vi "Write Max Redirects.vi"(8 "error in (no error)":errorcluster, 10 "max redirects (-1 = no limit)":i32=-1, 11 "REST Client in":refnum<class "REST Client.lvclass">) -> (0 "error out":errorcluster, 3 "REST Client out":refnum<class "REST Client.lvclass">)   [LabVIEW 2020, in "REST Client.lvlib" / "REST Client.lvclass"]
uses:
  REST Client.lvclass
  REST Client.lvclass/REST Client.ctl
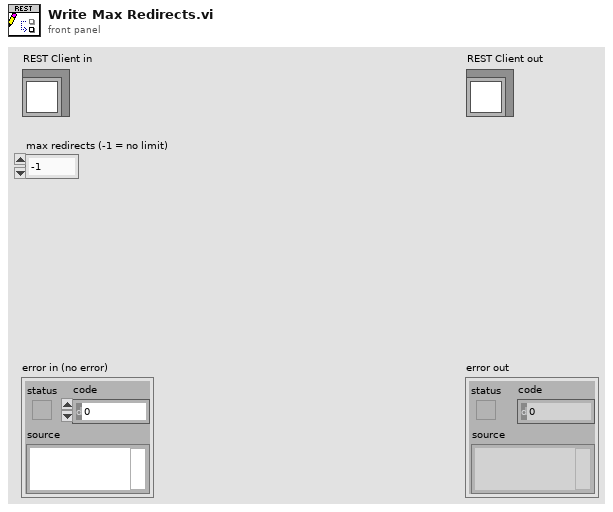
[diagram p1: front panel]
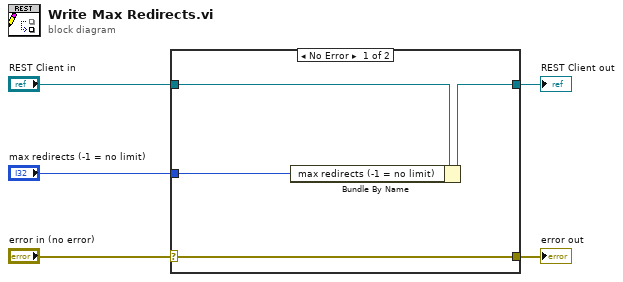
[diagram p0: block diagram]
diagram:
  n1 = case shown="No Error" "error in (no error)" {
    selector: "error in (no error)" -> [w9 w10]
    tunnel: [w9 w10] -> w4
    tunnel: [w7 w11] -> w2
    tunnel: "REST Client in" -> [w8 w11]
    tunnel: "max redirects (-1 = no limit)" -> [w6 _]
    frame No Error {
      n2 = Bundle By Name(cluster=w8, "max redirects (-1 = no limit)"=w6) -> (w7:refnum<class "REST Client.lvclass">)
    }
    frame Error {
    }
  }
  "error out" <- w4
  "REST Client out" <- w2
